vi "6b.vi"() -> ()   [LabVIEW 2015]
panel:
  in  "Cluster":cluster{"String":string, "Data":dbl[][]}={"String"="", "Data"=[[0.0, 0.18812375309361767, 0.3740231207291591, 0.5555058672704027, 0.7304435612665703, 0.8968022466674207, 1.0526716586133669, 1.1962925343408621, 1.3260815996037305, 1.4406538474450166, 1.538841768587627, 1.6197112404773788, 1.6825738343569605, 1.7269953558496833, 1.7528004935044779, 1.760073510670101, 1.7491549779680344, 1.7206346055458783, 1.6753402952418084, 1.6143235918169396, 1.5388417685876266, 1.4503368352303463, 1.3504118034133665, 1.2408045884793326, 1.123359961992576, 1.0000000000000007, 0.8726934948639677, 0.7434248141496237, 0.6141626980440116, 0.4868294870269171, 0.36327126400268184, 0.24522937995956395, 0.13431380969023166, 0.03197875454184962, -0.06049912696400295, -0.14203952192020497, -0.21177400795289814, -0.2690581010068591, -0.31347962249958217, -0.3448632609799984, -0.36327126400268017, -0.3690002574870229, -0.3625742514003001, -0.34473395121071715, -0.3164225532440117, -0.2787682579175269, -0.23306378693686225, -0.18074323809895523, -0.12335665360055248, -0.06254271403499326, -2.342906684632551e-15, 0.06254271403498819, 0.12335665360054807, 0.1807432380989511, 0.23306378693685822, 0.2787682579175238, 0.3164225532440093, 0.3447339512107155, 0.3625742514002992, 0.3690002574870229, 0.36327126400268106, 0.3448632609800002, 0.31347962249958505, 0.2690581010068628, 0.2117740079529028, 0.14203952192021063, 0.060499126964010164, -0.03197875454184307, -0.13431380969022366, -0.24522937995955496, -0.3632712640026733, -0.48682948702690765, -0.6141626980440016, -0.7434248141496149, -0.8726934948639604, -0.9999999999999943, -1.1233599619925714, -1.2408045884793277, -1.350411803413363, -1.450336835230344, -1.5388417685876252, -1.6143235918169394, -1.6753402952418088, -1.720634605545879, -1.7491549779680347, -1.760073510670101, -1.7528004935044776, -1.7269953558496822, -1.6825738343569583, -1.619711240477375, -1.5388417685876221, -1.4406538474450095, -1.3260815996037234, -1.196292534340853, -1.0526716586133558, -0.8968022466674075, -0.7304435612665547, -0.5555058672703851, -0.37402312072913946, -0.18812375309359874, 2.058151826050958e-14, 0.18812375309363966, 0.37402312072918226, 0.5555058672704266, 0.7304435612665945, 0.896802246667445, 1.0526716586133884, 1.196292534340883, 1.3260815996037503, 1.4406538474450343, 1.5388417685876428, 1.619711240477392, 1.6825738343569707, 1.7269953558496898, 1.7528004935044812, 1.7600735106701006, 1.7491549779680304, 1.7206346055458703, 1.6753402952417964, 1.6143235918169236, 1.5388417685876061, 1.4503368352303234, 1.35041180341334, 1.2408045884793029, 1.1233599619925434, 0.9999999999999651, 0.8726934948639306, 0.743424814149585, 0.6141626980439736, 0.48682948702687673, 0.3632712640026434, 0.24522937995952498, 0.1343138096901958, 0.031978754541817644, -0.06049912696403403, -0.1420395219202314, -0.21177400795292212, -0.2690581010068779, -0.31347962249959704, -0.3448632609800082, -0.36327126400268483, -0.3690002574870227, -0.36257425140029514, -0.3447339512107072, -0.3164225532439976, -0.2787682579175082, -0.23306378693684013, -0.1807432380989309, -0.12335665360052503, -0.06254271403496459, 2.8054327524257294e-14, 0.0625427140350182, 0.12335665360057807, 0.18074323809897855, 0.23306378693688276, 0.27876825791754567, 0.31642255324402624, 0.344733951210728, 0.3625742514003058, 0.36900025748702314, 0.3632712640026744, 0.34486326097998665, 0.3134796224995632, 0.2690581010068339, 0.21177400795286538, 0.142039521920166, 0.06049912696395621, -0.03197875454190191, -0.13431380969028817, -0.24522937995962746, -0.3632712640027481, -0.4868294870269889, -0.6141626980440849, -0.7434248141497006, -0.8726934948640435, -1.0000000000000737, -1.1233599619926493, -1.2408045884794014, -1.3504118034134325, -1.450336835230405, -1.5388417685876796, -1.6143235918169838, -1.6753402952418424, -1.720634605545903, -1.7491549779680473, -1.7600735106701022, -1.752800493504467, -1.726995355849659, -1.6825738343569236, -1.6197112404773275, -1.538841768587564, -1.4406538474449422, -1.3260815996036428, -1.1962925343407647, -1.0526716586132567, -0.8968022466673031, -0.7304435612664418, -0.5555058672702697, -0.3740231207290231, -0.18812375309347495, 1.4241537636683343e-13, 0.18812375309376345, 0.3740231207293012, 0.5555058672705445, 0.7304435612667051, 0.8968022466675469, 1.0526716586134877, 1.1962925343409716, 1.326081599603831, 1.4406538474451032, 1.538841768587702, 1.6197112404774385, 1.6825738343570047, 1.7269953558497129, 1.7528004935044919, 1.7600735106700993, 1.7491549779680176, 1.720634605545846, 1.6753402952417618, 1.6143235918168801, 1.5388417685875528, 1.4503368352302624, 1.3504118034132706, 1.2408045884792294, 1.1233599619924635, 0.9999999999998839, 0.8726934948638492, 0.7434248141495011, 0.6141626980438903, 0.48682948702679546, 0.36327126400256515, 0.24522937995945082, 0.13431380969012674, 0.03197875454175447, -0.06049912696409043, -0.14203952192028035, -0.2117740079529632, -0.26905810100691085, -0.3134796224996216, -0.3448632609800243, -0.36327126400269294, -0.3690002574870225, -0.3625742514002872, -0.3447339512106922, -0.31642255324397617, -0.2787682579174811, -0.2330637869368083, -0.1807432380988937, -0.12335665360048664, -0.06254271403492455, 6.866561355969858e-14, 0.06254271403505823, 0.12335665360061643, 0.18074323809901416, 0.23306378693691598, 0.2787682579175714, 0.31642255324404867, 0.3447339512107431, 0.36257425140031374, 0.36900025748702336, 0.3632712640026663, 0.3448632609799698, 0.31347962249953865, 0.26905810100680105, 0.21177400795282608, 0.14203952192011482, 0.06049912696389981, -0.03197875454196508, -0.13431380969035733, -0.24522937995970495, -0.36327126400282983, -0.4868294870270702, -0.6141626980441679, -0.7434248141497807, -0.8726934948641303, -1.0000000000001585, -1.1233599619927275, -1.240804588479475, -1.3504118034134973, -1.4503368352304689, -1.5388417685877327, -1.614323591817028, -1.675340295241877, -1.720634605545928, -1.7491549779680609, -1.7600735106701033, -1.7528004935044563, -1.7269953558496391, -1.6825738343568934, -1.6197112404772893, -1.5388417685875213, -1.4406538474448913, -1.326081599603588, -1.196292534340711, -1.052671658613202, -0.8968022466672445, -0.7304435612663942, -0.5555058672702199, -0.37402312072898214, -0.18812375309343865, 1.7898410618194527e-13, 0.18812375309378387, 0.3740231207293213, 0.555505867270559, 0.7304435612667092, 0.8968022466675509, 1.052671658613487, 1.1962925343409632, 1.3260815996038202, 1.4406538474450938, 1.5388417685876865, 1.619711240477426, 1.6825738343569956, 1.726995355849704, 1.7528004935044876, 1.7600735106700998, 1.7491549779680242, 1.7206346055458597, 1.6753402952417815, 1.6143235918169094, 1.5388417685875906, 1.4503368352303054, 1.3504118034133277, 1.2408045884792909, 1.1233599619925323, 0.9999999999999625, 0.8726934948639298, 0.7434248141495858, 0.6141626980439818, 0.48682948702688833, 0.36327126400265464, 0.2452293799595454, 0.13431380969021478, 0.031978754541840404, -0.06049912696401116, -0.14203952192021152, -0.21177400795290013, -0.26905810100686023, -0.31347962249958283, -0.3448632609799973, -0.3632712640026796, -0.3690002574870229, -0.36257425140030153, -0.34473395121071987, -0.3164225532440157, -0.2787682579175345, -0.2330637869368712, -0.18074323809896564, -0.12335665360056744, -0.06254271403500887, -1.862079284167817e-14, 0.06254271403496865, 0.12335665360052891, 0.18074323809893295, 0.2330637869368392, 0.27876825791750737, 0.31642255324399604, 0.3447339512107048, 0.36257425140029353, 0.3690002574870226, 0.3632712640026874, 0.3448632609800135, 0.31347962249960526, 0.2690581010068932, 0.21177400795294132, 0.14203952192025648, 0.060499126964067784, -0.03197875454177701, -0.1343138096901454, -0.24522937995947092, -0.3632712640025828, -0.4868294870268066, -0.6141626980438983, -0.743424814149509, -0.8726934948638463, -0.9999999999998809, -1.1233599619924608, -1.2408045884792172, -1.3504118034132593, -1.4503368352302495, -1.5388417685875373, -1.614323591816865, -1.67534029524175, -1.7206346055458357, -1.7491549779680113, -1.7600735106700989, -1.7528004935044983, -1.7269953558497266, -1.6825738343570271, -1.6197112404774727, -1.5388417685877447, -1.440653847445157, -1.3260815996038997, -1.1962925343410522, -1.052671658613576, -0.8968022466676557, -0.7304435612668202, -0.5555058672706649, -0.3740231207294408, -0.18812375309390553]]}
  out "Signals":dbl[][](graph)
  in  "# of record":i32=20
  out "Data record":i32
  in  "physical channels":tag="Dev1/ai0:2"
  in  "Sampling rate":dbl=10000.0
  in  "# of samples":i32=500
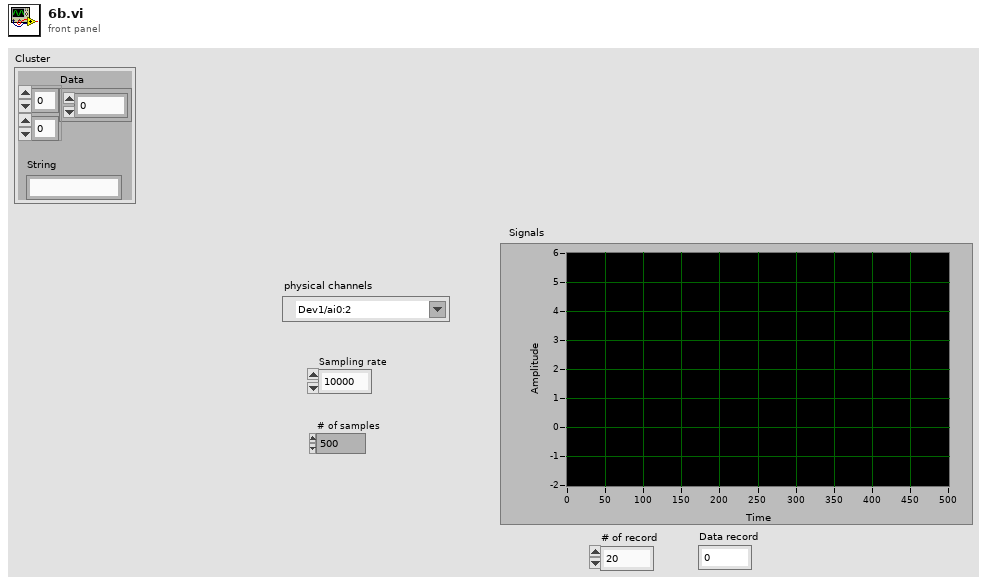
[diagram p1: front panel]
types:
  T1 = enum16{"open", "replace", "create", "open or create", "replace or create", "replace or create with confirmation"}
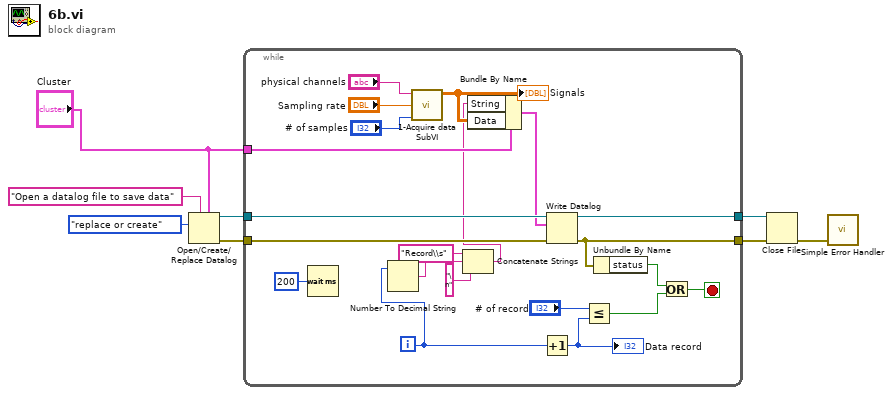
[diagram p0: block diagram]
diagram:
  n1 = Open/Create/Replace Datalog(5:"Cluster", 7:"Open a datalog file to save data" ("prompt"), 10:T1."replace or create" ("operation (0:open)")) -> (0:w8:errorcluster, 3:w6:refnum<k1>)  [unwired: 3 in, 1 out]
  n2 = while {
    tunnel: w8 -> [w29]
    tunnel: [w26] -> w7
    tunnel: w6 -> [w28]
    tunnel: [w27] -> w5
    tunnel: "Cluster" -> [w16]
    i -> [w13]
    stop <- w24 stop-if-true
    n3 = Wait (ms)(milliseconds to wait=u32 200) -> ()  [unwired: 1 out]
    n4 = Number To Decimal String(number=w13) -> (decimal integer string=w12:string)  [unwired: 1 in]
    n5 = call "1-Acquire data SubVI.vi"("# of samples/channel"="# of samples", "Sampling rate"="Sampling rate", "physical channels"="physical channels") -> ("data"=w15:dbl[][])  [unwired: 8 in]
    "Signals" <- w15
    n6 = Concatenate Strings("Record\\s" ("string"), w12, "\n" ("string")) -> (w9:string)
    n7 = Bundle By Name(cluster=w16, "String"=w9, "Data"=w15) -> (w14:cluster{"String":string, "Data":dbl[][]})
    n8 = Increment(x=w13) -> (x+1=w21:i32)
    "Data record" <- w21
    n9 = Write Datalog(4:w29, 6:w14, 7:w28) -> (0:w26:errorcluster, 3:w27:refnum<k1>)
    n10 = Less Or Equal?(x="# of record", y=w21) -> (x <= y?=w20:bool)
    n11 = Unbundle By Name(w26) -> ("status"=w25:bool)
    n12 = Or(x=w25, y=w20) -> (x .or. y?=w24:bool)
  }
  n13 = Close File(refnum=w5, error in=w7) -> (error out=w2:errorcluster)  [unwired: 1 out]
  n14 = call <vilib>:"Simple Error Handler.vi"("error in (no error)"=w2) -> ()  [unwired: 4 in, 5 out]
